vi "sync_alex_iteration.vi"(5 "frame number\n(starts with 1)":i32, 6 "error in":errorcluster, 7 "data value reference":refnum<data-value>, 8 "last frame (s)":dbl, 9 "DAQmx Task":refnum<k21>) -> (0 "error out":errorcluster, 1 "Stop?":bool, 2 "relative seconds 2":dbl, 3 "task out":refnum<k21>)   [LabVIEW 2023, in "NI DAQ.lvlib"]
uses:
  NI DAQ.lvlib
  Resources/Type Defs/sync device settings.ctl
  <vilib>/DAQmx/write.llb/DAQmx Write (Digital 1D Bool 1Chan 1Samp).vi
  <vilib>/DAQmx/miscellaneous.llb/DAQmx Fill In Error Info.vi
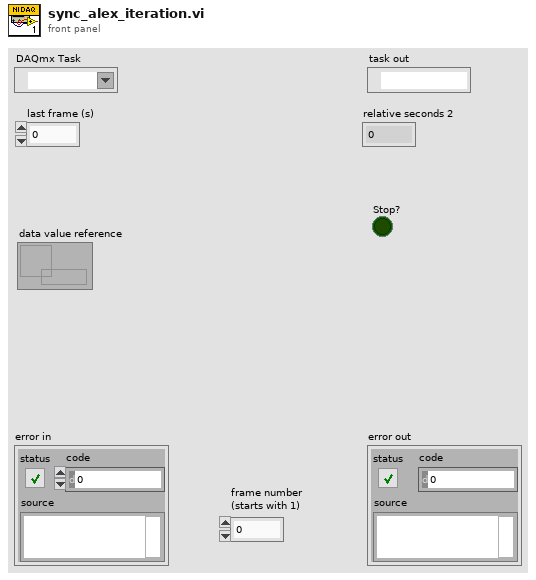
[diagram p1: front panel]
types:
  T1 = typedef "sync device settings.ctl" = cluster{"Interval (ms)":dbl, "ALEX":bool, "Shutter Enable":bool[], "Stream":bool, "Duty Cycle":dbl, "fluidics trigger frame":u16, "Frames to Skip":u32}
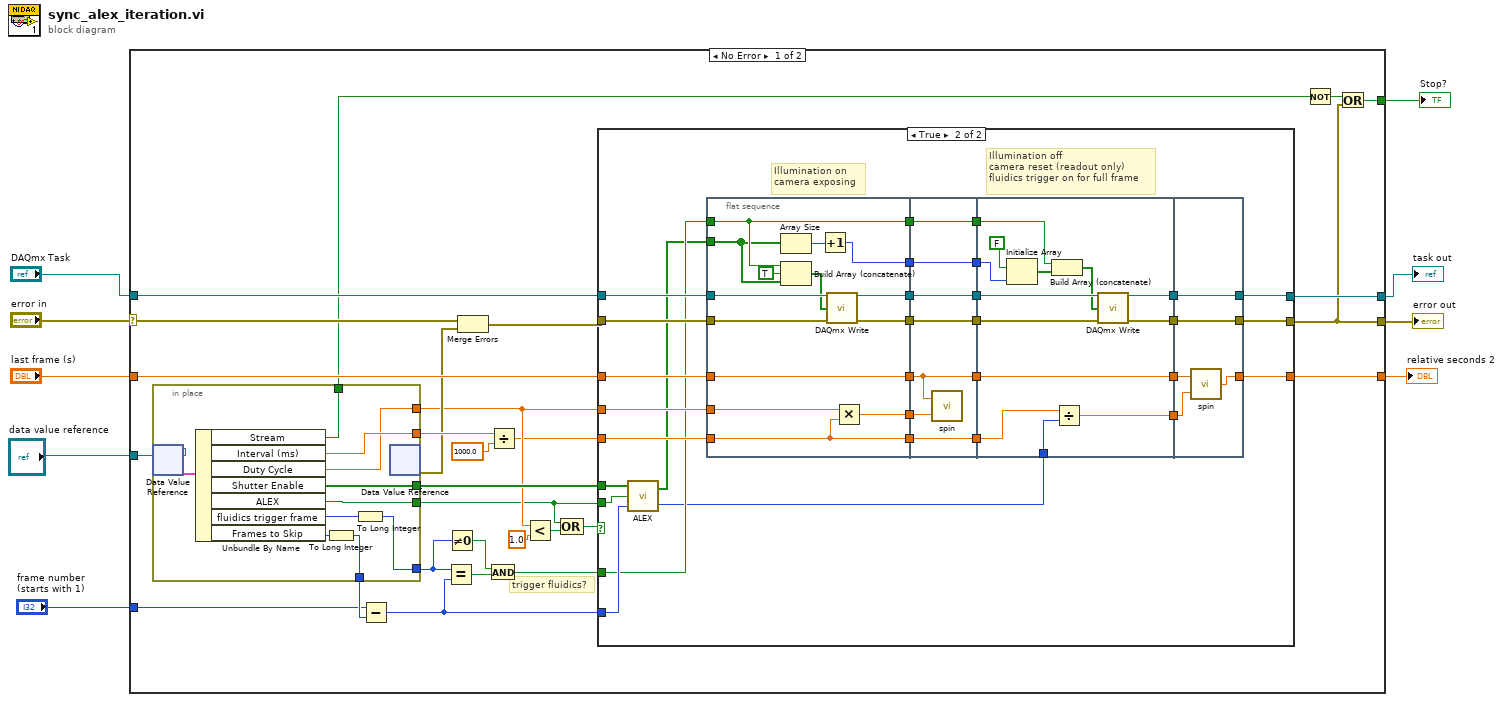
[diagram p0: block diagram]
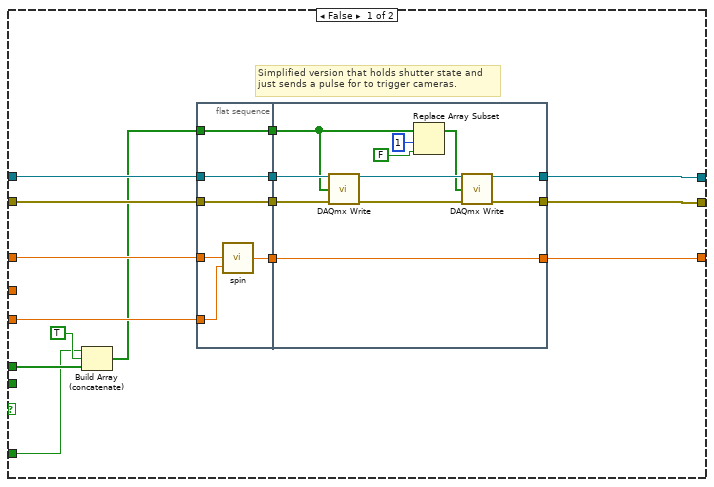
[diagram p2: hidden frame]
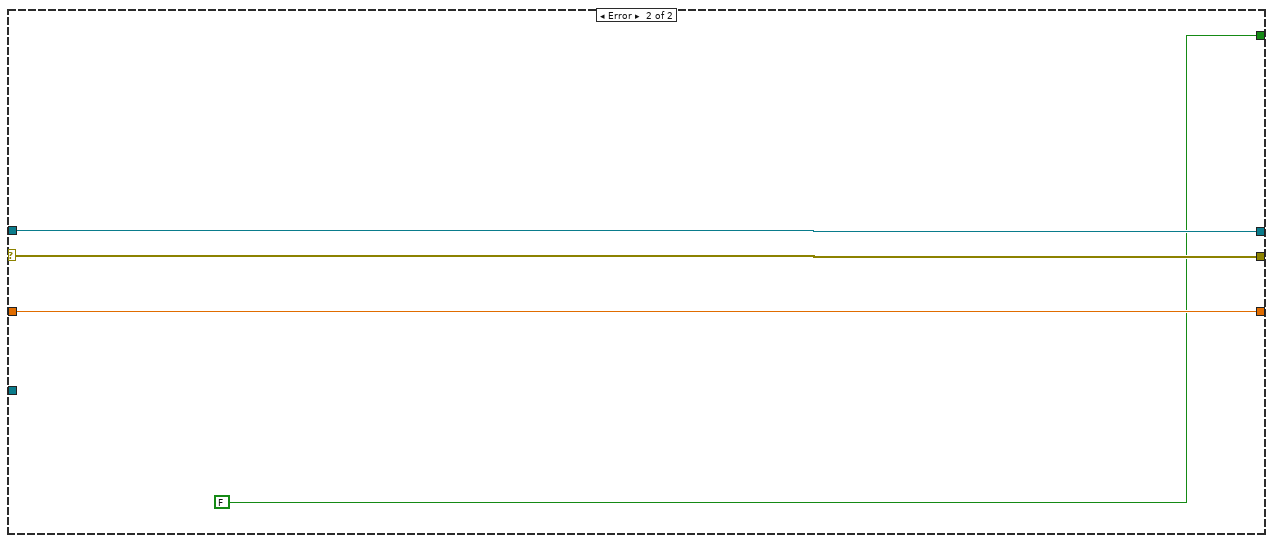
[diagram p3: hidden frame]
diagram:
  n1 = case shown="No Error" "error in" {
    selector: "error in" -> [w31 w151]
    tunnel: "DAQmx Task" -> [w37 w153]
    tunnel: [w36 w153] -> w8
    tunnel: [w19 w151] -> w7
    tunnel: "last frame (s)" -> [w35 w152]
    tunnel: [w34 w152] -> w5
    tunnel: "frame number\n(starts with 1)" -> [w10 _]
    tunnel: "data value reference" -> [w21 _]
    tunnel: [w29 FALSE] -> w2
    frame No Error {
      # "trigger fluidics?"
      n2 = in-place {
        in-place-border: [w46] -> w33
        in-place-border: [w47] -> w28
        in-place-border: [w45] -> w24
        in-place-border: [w42] -> w26
        in-place-border: [w38] -> w14
        in-place-border: [w43] -> w17
        in-place-border: [w40] -> w15
        n3 = in-place-dvr #1(w21) -> (w44:T1)  [unwired: 1 out]
        n4 = Unbundle By Name(w44) -> ("Stream"=w43:bool, "Interval (ms)"=w46:dbl, "Duty Cycle"=w42:dbl, "Shutter Enable"=w47:bool[], "ALEX"=w45:bool, "fluidics trigger frame"=w39:u16, "Frames to Skip"=w41:u32)
        n5 = To Long Integer(number=w41) -> (32bit integer=w40:i32)
        n6 = To Long Integer(number=w39) -> (32bit integer=w38:i32)
        n7 = in-place-dvr #1() -> (w27:errorcluster)  [unwired: 1 in, 1 out]
      }
      n8 = Subtract(x=w10, y=w15) -> (x-y=w16:i32)
      n9 = Equal?(x=w14, y=w16) -> (x = y?=w13:bool)
      n10 = Not Equal To 0?(x=w14) -> (x != 0?=w12:bool)
      n11 = Merge Errors(w31, w27) -> (w30:errorcluster)
      n12 = And(x=w12, y=w13) -> (x .and. y?=w11:bool)
      n13 = Divide(x=w33, y=1000.0) -> (x/y=w20:dbl)
      n14 = Less?(x=w26, y=1.0) -> (x < y?=w23:bool)
      n15 = Compound Arithmetic op=OR(w24, w23) -> (w22:bool)
      n16 = case shown="True" w22 {
        tunnel: w37 -> [w60 w100]
        tunnel: [w62 w93] -> w36
        tunnel: w35 -> [w55 w94]
        tunnel: [w53 w99] -> w34
        tunnel: w26 -> [_ w89]
        tunnel: w20 -> [w56 w90]
        tunnel: w30 -> [w59 w98]
        tunnel: [w61 w92] -> w19
        tunnel: w16 -> [_ w97]
        tunnel: w24 -> [_ w96]
        tunnel: w28 -> [w51 w95]
        tunnel: w11 -> [w50 w86]
        frame False {
          # "Simplified version that holds shutter state and\njust sends a pulse for to trigger cameras."
          n17 = Build Array (concatenate)(w50, TRUE, w51) -> (w49:bool[])
          n18 = flat-sequence {
            tunnel: w59 -> [w67]
            tunnel: w60 -> [w68]
            tunnel: [w68] -> w58
            tunnel: [w67] -> w57
            tunnel: w56 -> [w64]
            tunnel: w55 -> [w66]
            tunnel: [w65] -> w54
            tunnel: w49 -> [w63]
            tunnel: [w63] -> w48
            tunnel: [w79] -> w62
            tunnel: [w77] -> w61
            tunnel: w58 -> [w75]
            tunnel: w57 -> [w74]
            tunnel: w54 -> [w73]
            tunnel: [w73] -> w53
            tunnel: w48 -> [w69]
            frame #0 {
              n19 = call "spin.vi"("Interval"=w64, "relative seconds"=w66) -> ("relative seconds 2"=w65:dbl)
            }
            frame #1 {
              n20 = call-poly <vilib>:"DAQmx Write.vi"("task/channels in"=w75, "data"=w69, "error in"=w74) -> ("task out"=w78:refnum<k21>, "error out"=w76:errorcluster)  [unwired: 10 in, 1 out]
              n21 = Replace Array Subset(array=w69, new element=FALSE ("new element/subarray"), index=1) -> (w72:bool[])
              n22 = call-poly <vilib>:"DAQmx Write.vi"("task/channels in"=w78, "data"=w72, "error in"=w76) -> ("task out"=w79:refnum<k21>, "error out"=w77:errorcluster)  [unwired: 10 in, 1 out]
            }
          }
        }
        frame True {
          # "Illumination off\ncamera reset (readout only)\nfluidics trigger on for full frame"
          # "Illumination on\ncamera exposing"
          n23 = call "ALEX.vi"("Frame Number\n(starts with 1)"=w97, "ALEX?"=w96, "Shutter Enable"=w95) -> ("ALEX lines"=w80:i16, "Shutter State"=w85:bool[])
          n24 = flat-sequence {
            tunnel: [w123] -> w110
            tunnel: [w120] -> w109
            tunnel: [w121] -> w108
            tunnel: [w118] -> w107
            tunnel: w100 -> [w124]
            tunnel: w98 -> [w122]
            tunnel: w94 -> [w120]
            tunnel: w90 -> [w117]
            tunnel: w89 -> [w119]
            tunnel: [w117] -> w88
            tunnel: w86 -> [w114]
            tunnel: w85 -> [w113]
            tunnel: [w114] -> w83
            tunnel: [w111] -> w81
            tunnel: w110 -> [w131]
            tunnel: [w131] -> w106
            tunnel: w109 -> [w129]
            tunnel: [w129] -> w105
            tunnel: w108 -> [w130]
            tunnel: [w130] -> w104
            tunnel: w107 -> [w128]
            tunnel: w88 -> [w127]
            tunnel: [w127] -> w87
            tunnel: [w126] -> w84
            tunnel: w83 -> [w126]
            tunnel: [w125] -> w82
            tunnel: w81 -> [w125]
            tunnel: w106 -> [w143]
            tunnel: w105 -> [w140]
            tunnel: w104 -> [w142]
            tunnel: [w141] -> w103
            tunnel: [w144] -> w102
            tunnel: [w140] -> w101
            tunnel: [w133] -> w91
            tunnel: w87 -> [w134]
            tunnel: w84 -> [w138]
            tunnel: w82 -> [w136]
            tunnel: w80 -> [w132]
            tunnel: w103 -> [w146]
            tunnel: w102 -> [w147]
            tunnel: w101 -> [w149]
            tunnel: [w148] -> w99
            tunnel: [w147] -> w93
            tunnel: [w146] -> w92
            tunnel: w91 -> [w145]
            frame #0 {
              n25 = Array Size(array=w113) -> (size(s)=w112:i32)
              n26 = Build Array (concatenate)(w114, TRUE, w113) -> (w116:bool[])
              n27 = Increment(x=w112) -> (x+1=w111:i32)
              n28 = call-poly <vilib>:"DAQmx Write.vi"("task/channels in"=w124, "data"=w116, "error in"=w122) -> ("task out"=w123:refnum<k21>, "error out"=w121:errorcluster)  [unwired: 10 in, 1 out]
              n29 = Multiply(x=w119, y=w117) -> (x*y=w118:dbl)
            }
            frame #1 {
              n30 = call "spin.vi"("Interval"=w128, "relative seconds"=w129) -> ()  [unwired: 1 out]
            }
            frame #2 {
              n31 = Initialize Array(FALSE, w136) -> (w135:bool[])
              n32 = Build Array (concatenate)(w138, w135) -> (w139:bool[])
              n33 = Divide(x=w134, y=w132) -> (x/y=w133:dbl)
              n34 = call-poly <vilib>:"DAQmx Write.vi"("task/channels in"=w143, "data"=w139, "error in"=w142) -> ("task out"=w144:refnum<k21>, "error out"=w141:errorcluster)  [unwired: 10 in, 1 out]
            }
            frame #3 {
              n35 = call "spin.vi"("Interval"=w145, "relative seconds"=w149) -> ("relative seconds 2"=w148:dbl)
            }
          }
        }
      }
      n36 = Not(x=w17) -> (.not. x?=w18:bool)
      n37 = Or(x=w18, y=w19) -> (x .or. y?=w29:bool)
    }
    frame Error {
    }
  }
  "task out" <- w8
  "error out" <- w7
  "relative seconds 2" <- w5
  "Stop?" <- w2
